vi "Read SecurityKey.vi"(8 "error in (no error)":errorcluster, 11 "BB-Series in":refnum<class "BB-Series.lvclass">) -> (0 "error out":errorcluster, 2 "SecurityKey":bool[](array[boolean]), 3 "BB-Series out":refnum<class "BB-Series.lvclass">)   [LabVIEW 2021, in "BB-Series.lvclass"]
uses:
  BB-Series.lvclass
  BB-Series.lvclass/BB-Series.ctl
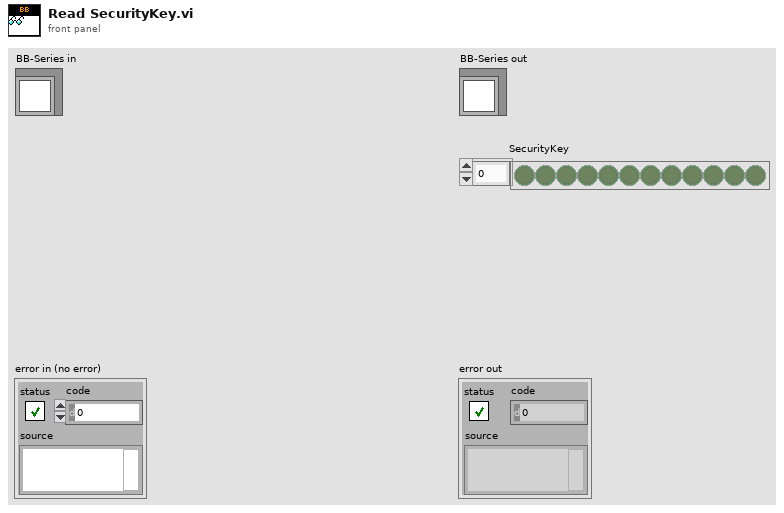
[diagram p1: front panel]
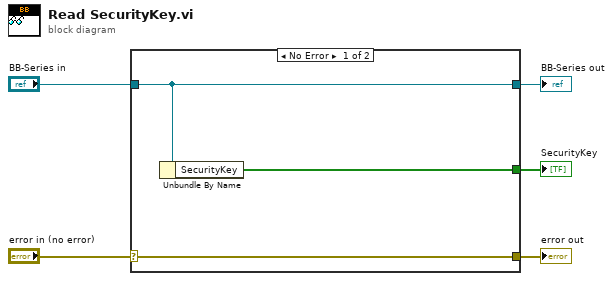
[diagram p0: block diagram]
diagram:
  n1 = case shown="No Error" "error in (no error)" {
    selector: "error in (no error)" -> [w8 w9]
    tunnel: [w8 w9] -> w4
    tunnel: [w7 w10] -> w2
    tunnel: "BB-Series in" -> [w7 w10]
    tunnel: [w6 _] -> w1
    frame No Error {
      n2 = Unbundle By Name(w7) -> ("SecurityKey"=w6:bool[])
    }
    frame Error {
    }
  }
  "error out" <- w4
  "BB-Series out" <- w2
  "SecurityKey" <- w1
